vi "arreglosCluster2.vi"() -> ()   [LabVIEW 2011]
uses:
  ControlArregloCluste2.ctl
panel:
  out "Array":T1(array[cluster]) {"velocidad 3" scale=0.0..180.0; "velocidad 2" scale=0.0..180.0; "velocidad1" scale=0.0..180.0}
  # "se tiene que ingresar  las tres velocidades de cada elemento del arreglo \nluego se debera de obtener el promedio de cada uno de los elementos del arreglo\n\nIniciar arreglo, rellenar arreglo , obtener promedio,finalizar."
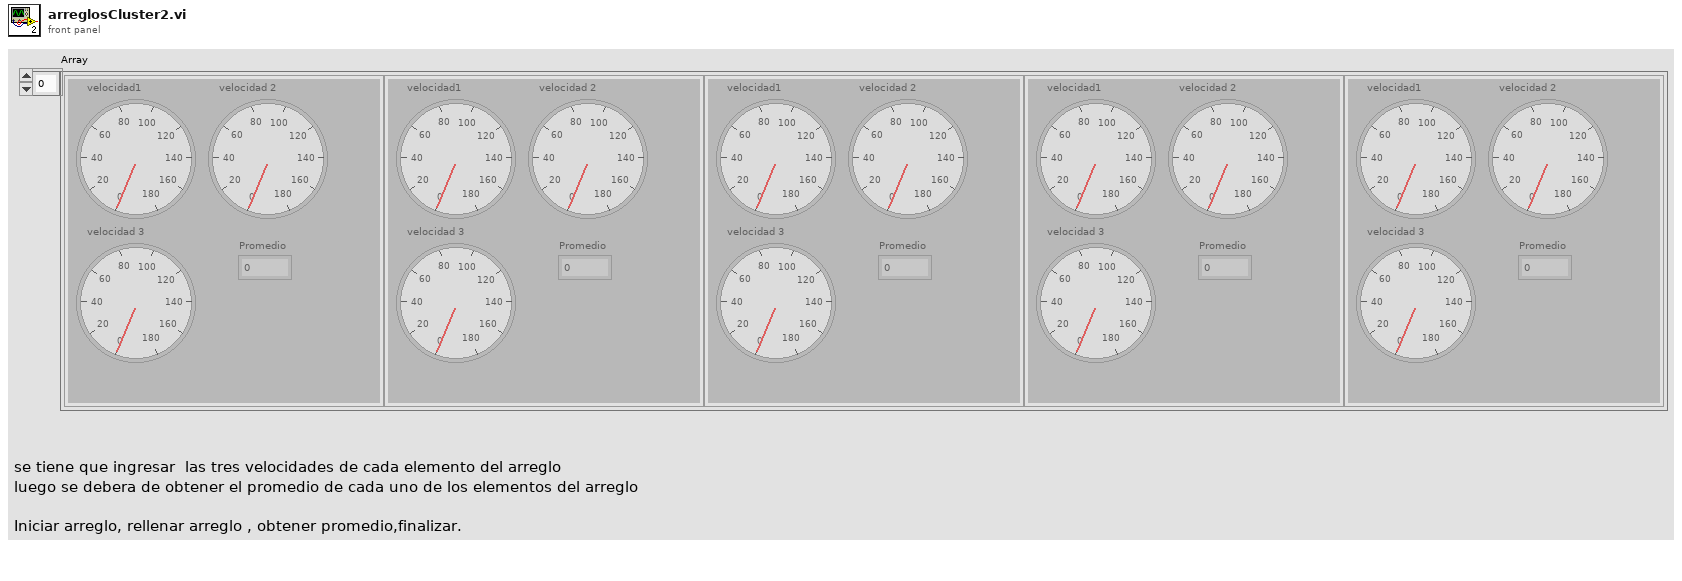
[diagram p1: front panel]
types:
  T1 = cluster{"velocidad1":dbl, "velocidad 2":dbl, "velocidad 3":dbl, "Promedio":dbl}[]
  T2 = typedef "ControlArregloCluste2.ctl" = enum16{"inicializar Arreglo", "rellenar arreglo", "calcular promedio", "Finalizar"}
  T3 = cluster{"velocidad1":dbl, "velocidad 2":dbl, "velocidad 3":dbl, "Promedio":dbl}
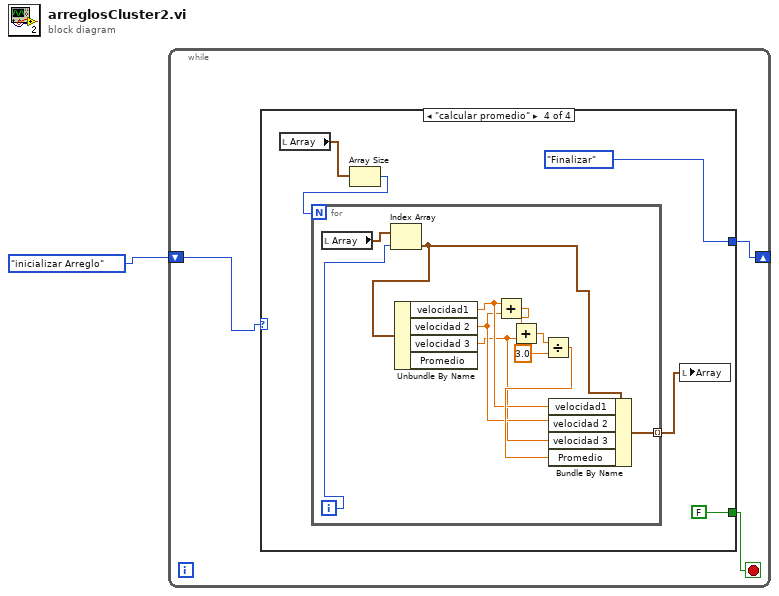
[diagram p0: block diagram]
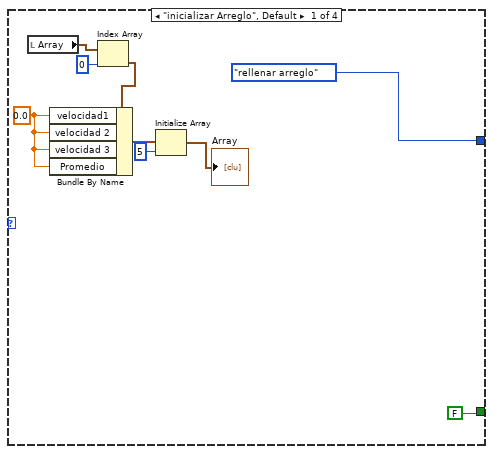
[diagram p2: hidden frame]
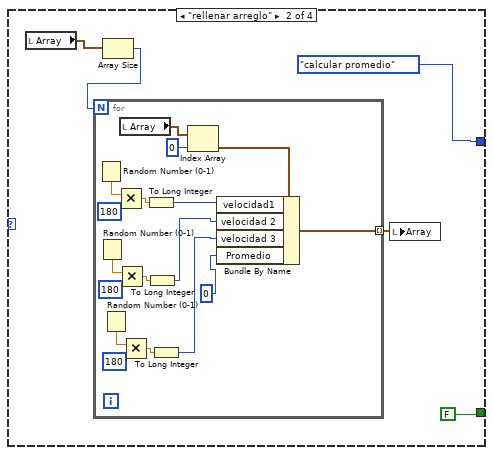
[diagram p3: hidden frame]
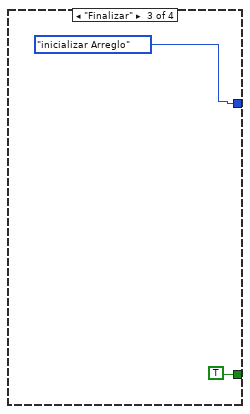
[diagram p4: hidden frame]
diagram:
  n1 = while {
    shift-right: [w3] -> _
    shift-left: ControlArregloCluste2."inicializar Arreglo" -> [w4]
    stop <- w2 stop-if-true
    n2 = case shown="\"calcular promedio\"" w4 {
      tunnel: [ControlArregloCluste2."rellenar arreglo" ControlArregloCluste2."calcular promedio" ControlArregloCluste2."inicializar Arreglo" ControlArregloCluste2."Finalizar"] -> w3
      tunnel: [FALSE FALSE TRUE FALSE] -> w2
      frame "inicializar Arreglo", Default {
        w7 = 0.0 ("velocidad1")
        n3 = local read "Array"() -> (w13:T1)
        n4 = Index Array "Index Array"(array=w13, index=0) -> (element=w11:T3)
        n5 = Bundle By Name(cluster=w11, "velocidad1"=w7, "velocidad 2"=w7, "velocidad 3"=w7, "Promedio"=w7) -> (w10:T3)
        n6 = Initialize Array "Initialize Array"(w10, 5 ("dimension size")) -> (→"Array":T1)
      }
      frame "rellenar arreglo" {
        n7 = local read "Array"() -> (w17:T1)
        n8 = Array Size(array=w17) -> (size(s)=w18:i32)
        n9 = for {
          N: w18 -> [_]
          tunnel: [w20] -> w16 mode=indexing
          n10 = Random Number (0-1)() -> (number: 0 to 1=w32:dbl)
          n11 = Random Number (0-1)() -> (number: 0 to 1=w26:dbl)
          n12 = Random Number (0-1)() -> (number: 0 to 1=w24:dbl)
          n13 = Multiply(x=w32, y=180) -> (x*y=w30:dbl)
          n14 = Multiply(x=w26, y=180) -> (x*y=w28:dbl)
          n15 = local read "Array"() -> (w35:T1)
          n16 = Multiply(x=w24, y=180) -> (x*y=w22:dbl)
          n17 = To Long Integer(number=w30) -> (32bit integer=w29:i32)
          n18 = To Long Integer(number=w28) -> (32bit integer=w25:i32)
          n19 = To Long Integer(number=w22) -> (32bit integer=w21:i32)
          n20 = Index Array(array=w35, index=0) -> (element=w33:T3)
          n21 = Bundle By Name(cluster=w33, "velocidad1"=w29, "velocidad 2"=w25, "velocidad 3"=w21, "Promedio"=0) -> (w20:T3)
        }
        n22 = local write "Array"(w16) -> ()
      }
      frame "Finalizar" {
      }
      frame "calcular promedio" {
        n23 = local read "Array"() -> (w42:T1)
        n24 = Array Size(array=w42) -> (size(s)=w41:i32)
        n25 = for {
          N: w41 -> [_]
          tunnel: [w43] -> w40 mode=indexing
          i -> [w52]
          n26 = local read "Array"() -> (w53:T1)
          n27 = Index Array "Index Array"(array=w53, index=w52) -> (element=w48:T3)
          n28 = Unbundle By Name "Unbundle By Name"(w48) -> ("velocidad1"=w46:dbl, "velocidad 2"=w45:dbl, "velocidad 3"=w44:dbl)  [unwired: 1 out]
          n29 = Add(x=w46, y=w45) -> (x+y=w51:dbl)
          n30 = Add(x=w51, y=w44) -> (x+y=w50:dbl)
          n31 = Divide(x=w50, y=3.0) -> (x/y=w47:dbl)
          n32 = Bundle By Name(cluster=w48, "velocidad1"=w46, "velocidad 2"=w45, "velocidad 3"=w44, "Promedio"=w47) -> (w43:T3)
        }
        n33 = local write "Array"(w40) -> ()
      }
    }
  }
